vi "UTILITY Double Array to String Array.vi"(11 "Hex Array Out":dbl[](array[numeric])) -> (3 "Array":string[](array[string]))   [LabVIEW 2016]
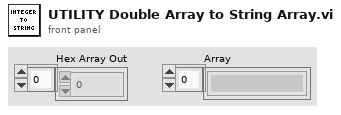
[diagram p1: front panel]
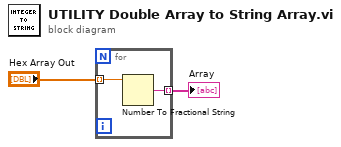
[diagram p0: block diagram]
diagram:
  n1 = for {
    tunnel: "Hex Array Out" -> [w4] mode=indexing
    tunnel: [w3] -> w2 mode=indexing
    n2 = Number To Fractional String(number=w4) -> (F-format string=w3:string)  [unwired: 3 in]
  }
  "Array" <- w2
